vi "DecodifyFrequency(Array).vi"(1 "Array 2":u32[](array[numeric])) -> (0 "Array":dbl[](array[numeric]) min=60.0 max=90.0 step=0.1)   [LabVIEW 2017, in "AODControl.lvlib"]
uses:
  AODControl.lvlib
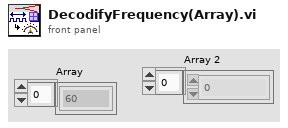
[diagram p1: front panel]
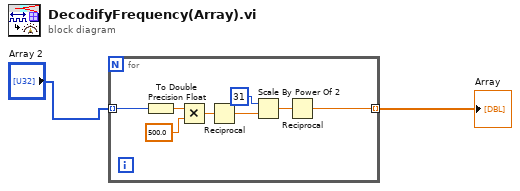
[diagram p0: block diagram]
diagram:
  n1 = for {
    tunnel: "Array 2" -> [w8] mode=indexing
    tunnel: [w3] -> w1 mode=indexing
    n2 = To Double Precision Float(number=w8) -> (double precision float=w7:dbl)
    n3 = Multiply(x=w7, y=500.0) -> (x*y=w6:dbl)
    n4 = Reciprocal(x=w6) -> (1/x=w5:dbl)
    n5 = Scale By Power Of 2(n=i16 31, x=w5) -> (x*2^n=w4:dbl)
    n6 = Reciprocal(x=w4) -> (1/x=w3:dbl)
  }
  "Array" <- w1
